vi "TDMS Remove Redundant System Fields From Group.vi"(1 "Fields In":T1[](array[typedef])) -> (0 "Fields Out":T1[](array[typedef]))   [LabVIEW 2011]
uses:
  database/Fields/Field Record.ctl
  database/Fields/Field DataTypes.ctl
  database/Fields/Field NextItem.ctl
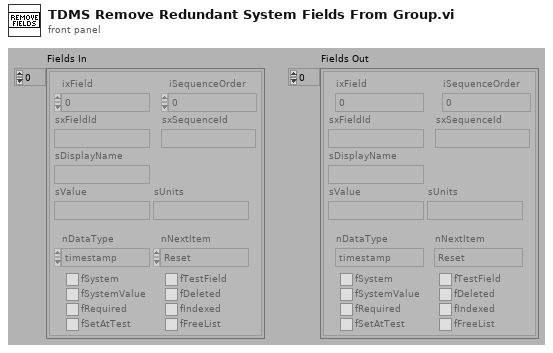
[diagram p1: front panel]
types:
  T1 = typedef "Field Record.ctl" = cluster{"ixField":i32, "iSequenceOrder":i32, "sxFieldId":string, "sxSequenceId":string, "sDisplayName":string, "sValue":string, "sUnits":string, "nDataType":T2, "nNextItem":T3, "fSystem":bool, "fSystemValue":bool, "fRequired":bool, "fSetAtTest":bool, "fTestField":bool, "fDeleted":bool, "fIndexed":bool, "fFreeList":bool}
  T2 = typedef "Field DataTypes.ctl" = enum32{"text", "numeric", "list", "timestamp", "boolean"}
  T3 = typedef "Field NextItem.ctl" = enum32{"Reset", "Retain", "Auto-Increment"}
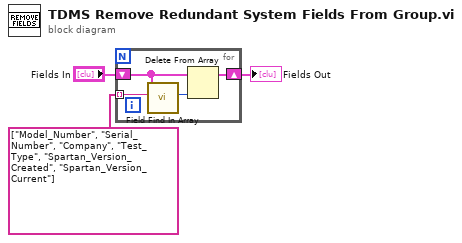
[diagram p0: block diagram]
diagram:
  n1 = for {
    shift-right: [w6] -> w2
    shift-left: "Fields In" -> [w7]
    tunnel: string[] ["Model_Number", "Serial_Number", "Company", "Test_Type", "Spartan_Version_Created", "Spartan_Version_Current"] -> [w4] mode=indexing
    n2 = call "Field Find In Array.vi"("FieldID or Display Name(\"\")"=w4, "Field Array"=w7) -> ("Index"=w5:i32)  [unwired: 1 in, 8 out]
    n3 = Delete From Array(array=w7, index=w5) -> (array with subset deleted=w6:T1[])  [unwired: 1 in, 1 out]
  }
  "Fields Out" <- w2
